vi "Page_Version_Write.vi"(6 "ctlReferences":T1, 8 "error in (no error)":errorcluster, 11 "Class in":refnum<class "IB_MSI.lvclass">) -> (0 "error out":errorcluster, 3 "Class out":refnum<class "IB_MSI.lvclass">)   [LabVIEW 2020, in "IB_MSI.lvclass"]
uses:
  <vilib>/AppBuilder/IB_Classes/MSI/IB_MSI.lvclass
  <resource>/Framework/Providers/Builds/Installer/Pages/controls/IB_UI_Page_Version_Info_References.ctl
  <resource>/Framework/Providers/Builds/Installer/CDK_sTypeDef_ProductVersion.ctl
  <vilib>/AppBuilder/IB_Classes/MSI/IB_MSI.lvclass/IB_MSI.ctl
  <vilib>/AppBuilder/IB_Classes/Installer/Installer.lvclass
panel:
  # "."
  # "."
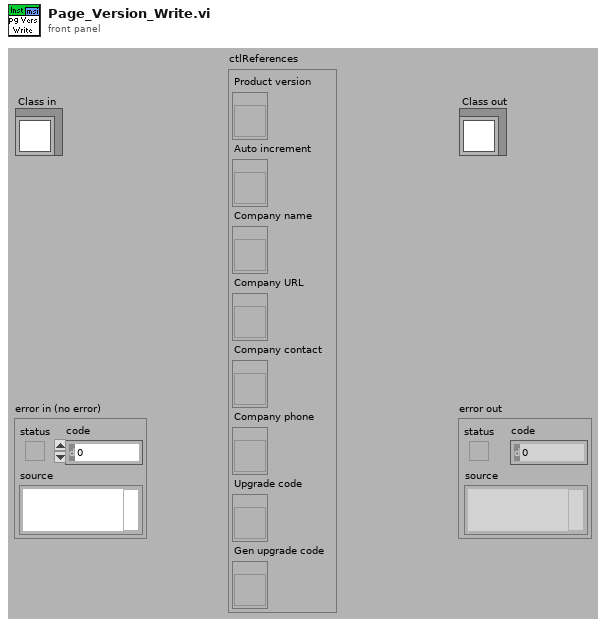
[diagram p1: front panel]
types:
  T1 = typedef "IB_UI_Page_Version_Info_References.ctl" = cluster{"Product version":refnum<vi>, "Auto increment":refnum<vi>, "Company name":refnum<vi>, "Company URL":refnum<vi>, "Company contact":refnum<vi>, "Company phone":refnum<vi>, "Upgrade code":refnum<vi>, "Gen upgrade code":refnum<vi>}
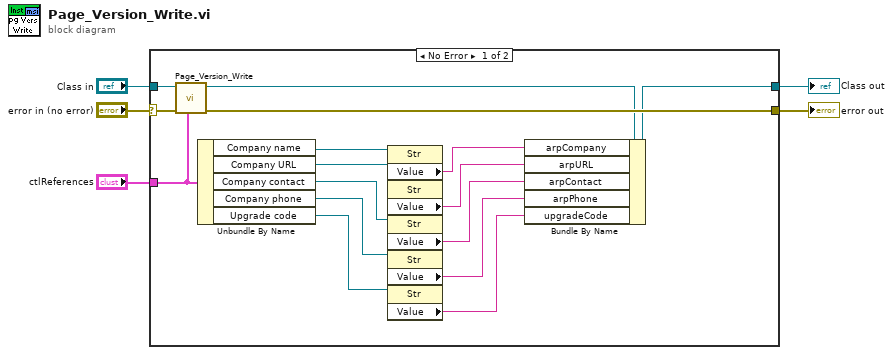
[diagram p0: block diagram]
diagram:
  n1 = case shown="No Error" "error in (no error)" {
    selector: "error in (no error)" -> [w19 w23]
    tunnel: [w18 w23] -> w4
    tunnel: [w15 w22] -> w2
    tunnel: "Class in" -> [w20 w22]
    tunnel: "ctlReferences" -> [w17 _]
    frame No Error {
      n2 = call-parent "Page_Version_Write.vi"("ctlReferences"=w17, "error in (no error)"=w19, "Class in"=w20) -> ("error out"=w18:errorcluster, "Class out"=w16:refnum<class "IB_MSI.lvclass">)  [unwired: 7 out]
      n3 = Unbundle By Name(w17) -> ("Company name"=w21:refnum<vi>, "Company URL"=w13:refnum<vi>, "Company contact"=w12:refnum<vi>, "Company phone"=w11:refnum<vi>, "Upgrade code"=w10:refnum<vi>)
      n4 = property class="Str"(reference=w21) -> ("Value"=w14:string)  [unwired: 1 in, 2 out]
      n5 = property class="Str"(reference=w13) -> ("Value"=w9:string)  [unwired: 1 in, 2 out]
      n6 = property class="Str"(reference=w12) -> ("Value"=w8:string)  [unwired: 1 in, 2 out]
      n7 = property class="Str"(reference=w11) -> ("Value"=w7:string)  [unwired: 1 in, 2 out]
      n8 = property class="Str"(reference=w10) -> ("Value"=w6:string)  [unwired: 1 in, 2 out]
      n9 = Bundle By Name(cluster=w16, "arpCompany"=w14, "arpURL"=w9, "arpContact"=w8, "arpPhone"=w7, "upgradeCode"=w6) -> (w15:refnum<class "IB_MSI.lvclass">)
    }
    frame Error {
    }
  }
  "error out" <- w4
  "Class out" <- w2
